vi "GetAllTaps.vi"(11 "Last Path":path) -> (0 "last tap":waveform(dbl)[](array[waveform]), 2 "files in pos":path[](array[path]), 3 "taps in pos":waveform(dbl)[](array[waveform]))   [LabVIEW 2022 SP3]
panel:
  out "filenames":string[](array[string])
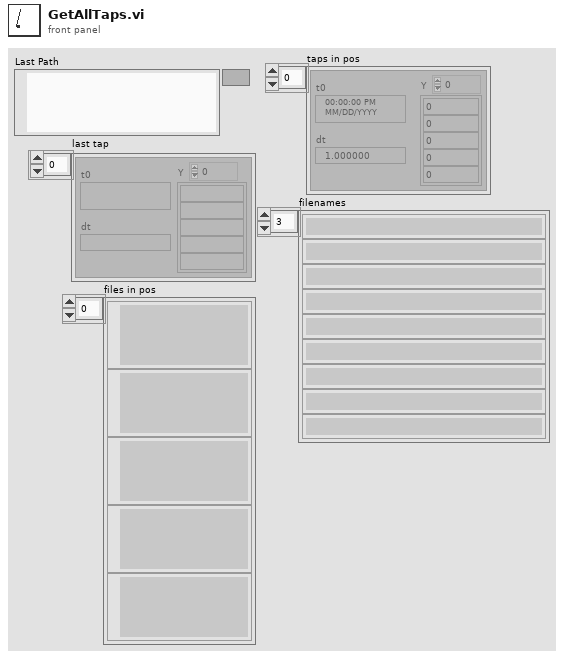
[diagram p1: front panel]
types:
  T1 = cluster{"Test":string, "Set":string, "Position":string, "Tap":string}
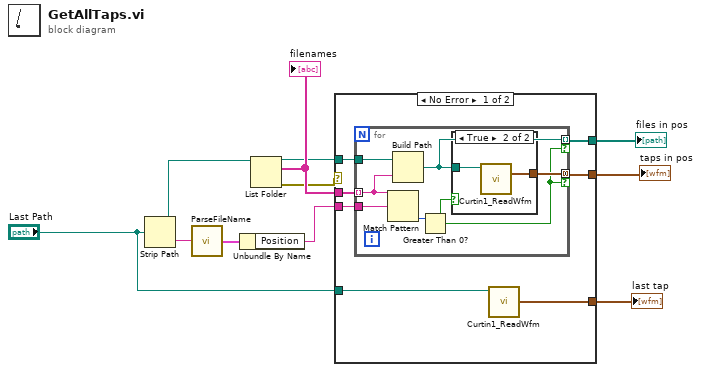
[diagram p0: block diagram]
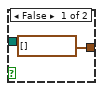
[diagram p2: hidden frame]
diagram:
  n1 = Strip Path(path="Last Path") -> (stripped path=w6:path, name=w5:string)
  n2 = call "ParseFileName.vi"("String in"=w5) -> ("Name"=w4:T1)  [unwired: 2 out]
  n3 = Unbundle By Name(w4) -> ("Position"=w3:string)
  n4 = List Folder(path=w6) -> (path out=w2:path, filenames=w11:string[], error out=w1:errorcluster)  [unwired: 3 in, 1 out]
  "filenames" <- w11
  n5 = case shown="No Error" w1 {
    tunnel: w11 -> [w18 _]
    tunnel: [w17 _] -> w10
    tunnel: [w16 _] -> w9
    tunnel: [w15 _] -> w8
    tunnel: "Last Path" -> [w14 _]
    tunnel: w3 -> [w13 _]
    tunnel: w2 -> [w12 _]
    frame No Error {
      n6 = for {
        tunnel: w18 -> [w23] mode=indexing
        tunnel: w13 -> [w25]
        tunnel: w12 -> [w22]
        tunnel: [w21] -> w17 mode=concatenating if=w19
        tunnel: [w20] -> w15 mode=indexing if=w19
        n7 = Match Pattern(string=w23, regular expression=w25) -> (offset past match=w24:i32)  [unwired: 1 in, 3 out]
        n8 = Build Path(base path=w22, name or relative path=w23) -> (appended path=w20:path)
        n9 = Greater Than 0?(x=w24) -> (x > 0?=w19:bool)
        n10 = case shown="True" w19 {
          tunnel: w20 -> [_ w28]
          tunnel: [waveform(dbl)[] [] ("all waveforms in record") w27] -> w21
          frame False {
          }
          frame True {
            n11 = call "Curtin1_ReadWfm.vi"("appended path"=w28) -> ("all waveforms in record"=w27:waveform(dbl)[])  [unwired: 9 in, 1 out]
          }
        }
      }
      n12 = call "Curtin1_ReadWfm.vi"("appended path"=w14) -> ("all waveforms in record"=w16:waveform(dbl)[])  [unwired: 9 in, 1 out]
    }
    frame Error {
    }
  }
  "taps in pos" <- w10
  "last tap" <- w9
  "files in pos" <- w8
